vi "Init.vi"(8 "error in (no error)":errorcluster, 10 "IConfigure":refnum<class "IConfigure.lvclass">, 11 "Camera Base in":refnum<class "Camera Base.lvclass">) -> (0 "error out":errorcluster, 3 "Camera Base out":refnum<class "Camera Base.lvclass">)   [LabVIEW 2023, in "Camera.lvlib" / "Camera Base.lvclass"]
uses:
  Camera Base.lvclass
  Interfaces/IConfigure/IConfigure.lvclass
  Camera Base.lvclass/Camera Base.ctl
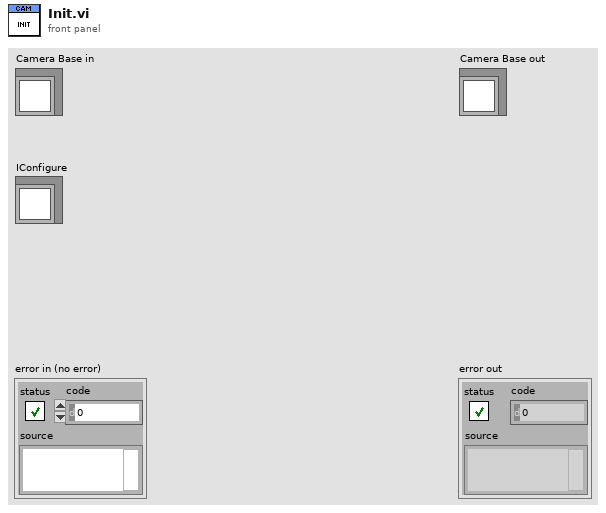
[diagram p1: front panel]
types:
  T1 = typedef "IMAQ Image.ctl" = refnum<image>
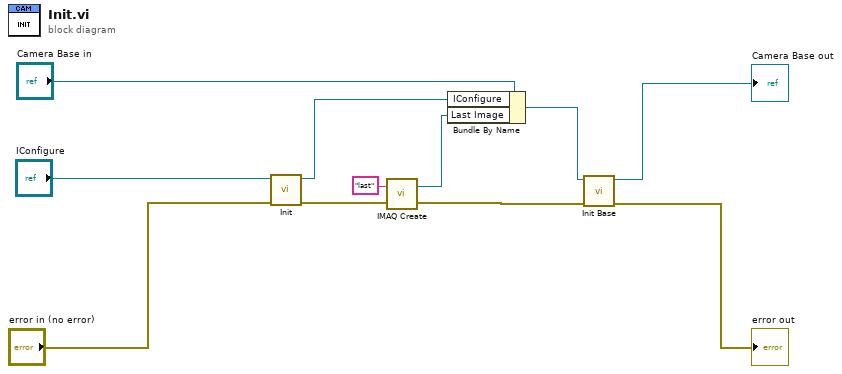
[diagram p0: block diagram]
diagram:
  n1 = call-dynamic "Init.vi"("error in"="error in (no error)", "IConfigure in"="IConfigure") -> ("error out"=w4:errorcluster, "IConfigure out"=w6:refnum<class "IConfigure.lvclass">)  [unwired: 8 in]
  n2 = call "IMAQ Create"("Image Name"="last", "error in (no error)"=w4) -> ("New Image"=w2:T1, "error out"=w3:errorcluster)  [unwired: 3 in]
  n3 = Bundle By Name(cluster="Camera Base in", "IConfigure"=w6, "Last Image"=w2) -> (w1:refnum<class "Camera Base.lvclass">)
  n4 = call-dynamic "Init Base.vi"("Error In"=w3, "object in"=w1) -> ("Error Out"=→"error out":errorcluster, "object out"=→"Camera Base out":refnum<class "Camera Base.lvclass">)  [unwired: 8 in]
